vi "Get Parity.vi"(8 "error in (no error)":errorcluster, 11 "RFFE RegRead Command in":refnum<class "RFFE RegRead Command.lvclass">) -> (0 "error out":errorcluster, 2 "Parity?":bool, 3 "RFFE RegRead Command out":refnum<class "RFFE RegRead Command.lvclass">)   [LabVIEW 2018, in "MIPI RFFE API.lvlib" / "RFFE RegRead Command.lvclass"]
uses:
  RFFE RegRead Command.lvclass
  RFFE RegRead Command.lvclass/RFFE RegRead Command.ctl
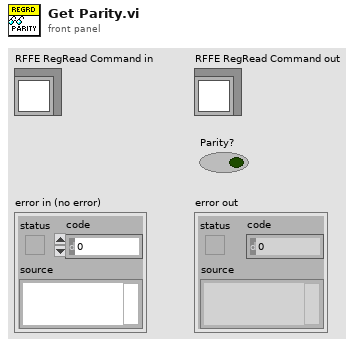
[diagram p1: front panel]
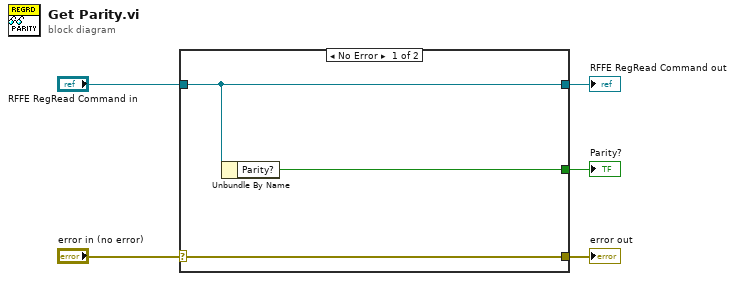
[diagram p0: block diagram]
diagram:
  n1 = case shown="No Error" "error in (no error)" {
    selector: "error in (no error)" -> [w8 w9]
    tunnel: [w8 w9] -> w4
    tunnel: [w7 w10] -> w2
    tunnel: "RFFE RegRead Command in" -> [w7 w10]
    tunnel: [w6 _] -> w1
    frame No Error {
      n2 = Unbundle By Name(w7) -> ("Parity?"=w6:bool)
    }
    frame Error {
    }
  }
  "error out" <- w4
  "RFFE RegRead Command out" <- w2
  "Parity?" <- w1
